vi "ElevatorPositions.vi"() -> ()   [LabVIEW 2014]
uses:
  <vilib>/Rock Robotics/Network Tables/SD Write Number.vi
panel:
  out "Elevator Req":dbl
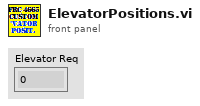
[diagram p1: front panel]
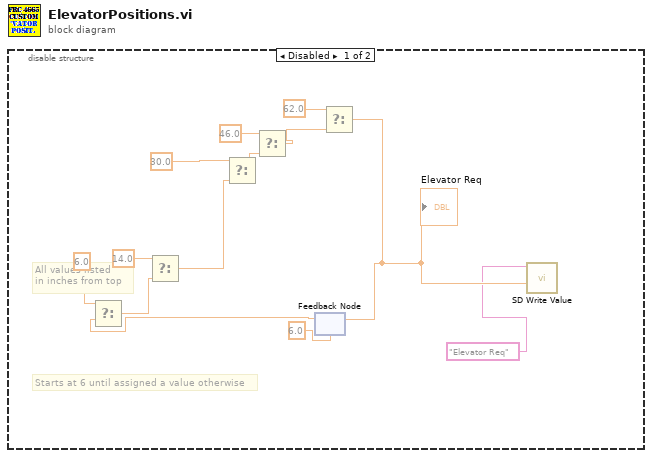
[diagram p0: block diagram]
diagram:
  n1 = disable-structure shown="Disabled" {
    frame Disabled {
      # "All values listed\nin inches from top"
      # "Starts at 6 until assigned a value otherwise"
      n2 = feedback #1(6.0 ("t")) -> (w2:dbl)
      n3 = Select(t=6.0, f=w2) -> (s? t:f=w3:dbl)  [unwired: 1 in]
      n4 = Select(t=14.0, f=w3) -> (s? t:f=w10:dbl)  [unwired: 1 in]
      n5 = Select(t=30.0, f=w10) -> (s? t:f=w11:dbl)  [unwired: 1 in]
      n6 = Select(t=46.0, f=w11) -> (s? t:f=w12:dbl)  [unwired: 1 in]
      n7 = Select(t=62.0, f=w12) -> (s? t:f=w5:dbl)  [unwired: 1 in]
      "Elevator Req" <- w5
      n8 = feedback-in #1(w5) -> ()
      n9 = call-poly <vilib>:"SD Write Value.vi"("Numeric"=w5, "Name"="Elevator Req") -> ()  [unwired: 8 in, 2 out]
    }
    frame Enabled {
    }
  }
